vi "Actuators Jog Forward.vi"(0 "Notifier Name":string, 2 "Wait to Finish":bool, 5 "Channel":i32[](array[numeric]), 11 "Error In":errorcluster) -> (4 "Notifier Name Out":string, 15 "Error Out":errorcluster)   [LabVIEW 2020]
uses:
  Actuators Controls/Actuators Note Type.ctl
  Actuators Controls/Actuators Actions.ctl
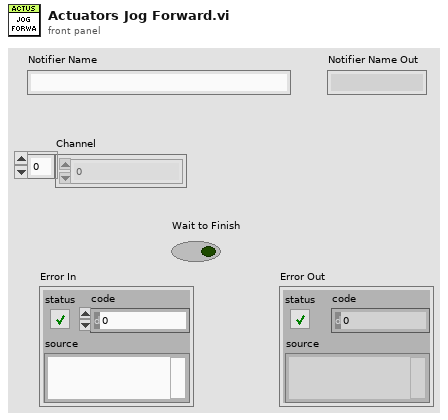
[diagram p1: front panel]
types:
  T1 = typedef "Actuators Note Type.ctl" = cluster{"Actions":T2, "Cmd Received ":bool, "Setpoint":dbl[], "Position":dbl[], "Channel":i32[], "Jog Step":dbl[], "Velocity":dbl[], "Acceleration":dbl[], "Status Bits":u32[], "Moving":bool[]}
  T2 = typedef "Actuators Actions.ctl" = enum16{"Nothing", "Get Position", "Get Acceleration", "Get Velocity", "Get Jog Step", "Set Acceleration", "Set Velocity", "Set Jog Step", "Move Absolute", "Move Relative", "Jog Forward", "Jog Reverse", "Halt", "Quit"}
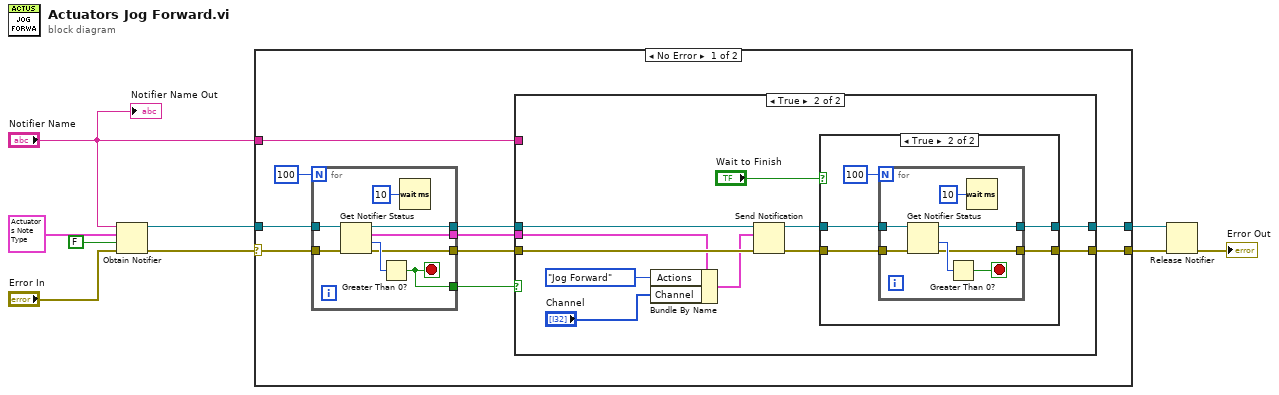
[diagram p0: block diagram]
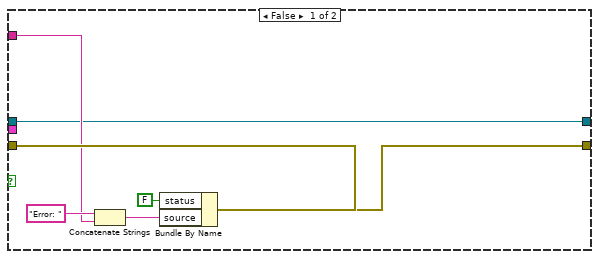
[diagram p2: hidden frame]
diagram:
  n1 = Obtain Notifier(name (unnamed)="Notifier Name", notification data type=T1 {"Actions"=enum."Nothing", "Cmd Received "=FALSE, "Setpoint"=[], "Position"=[], "Channel"=[], "Jog Step"=[], "Velocity"=[], "Acceleration"=[], "Status Bits"=[], "Moving"=[]} ("Actuators Note"), create if not found? (T)=FALSE, error in (no error)="Error In") -> (notifier out=w5:refnum<notifier>, error out=w8:errorcluster)  [unwired: 1 out]
  n2 = case shown="No Error" w8 {
    selector: w8 -> [w17 w60]
    tunnel: w5 -> [w18 w61]
    tunnel: "Notifier Name" -> [w12 _]
    tunnel: [w11 w61] -> w4
    tunnel: [w10 w60] -> w3
    frame No Error {
      n3 = for {
        N: 100 -> [_]
        tunnel: [w58] -> w14
        tunnel: w18 -> [w59]
        tunnel: [w57] -> w15
        tunnel: w17 -> [w54]
        tunnel: [w53] -> w16
        tunnel: [w52] -> w13
        stop <- w53 stop-if-true
        n4 = Get Notifier Status(notifier=w59, error in (no error)=w54) -> (notifier out=w57:refnum<notifier>, current notification=w58:T1, # waiting=w56:i32, error out=w52:errorcluster)  [unwired: 1 out]
        n5 = Greater Than 0?(x=w56) -> (x > 0?=w53:bool)
        n6 = Wait (ms)(milliseconds to wait=u32 10) -> ()  [unwired: 1 out]
      }
      n7 = case shown="True" w16 {
        tunnel: w15 -> [w21 w37]
        tunnel: w14 -> [_ w28]
        tunnel: w13 -> [w26 w36]
        tunnel: w12 -> [w22 _]
        tunnel: [w21 w32] -> w11
        tunnel: [w20 w33] -> w10
        frame False {
          n8 = Concatenate Strings("Error: " ("source"), w22) -> (w23:string)
          n9 = Bundle By Name(cluster=w26, "status"=FALSE, "source"=w23) -> (w20:errorcluster)
        }
        frame True {
          n10 = Bundle By Name(cluster=w28, "Actions"=Actuators_Actions."Jog Forward", "Channel"="Channel") -> (w29:T1)
          n11 = Send Notification(notification=w29, notifier=w37, error in (no error)=w36) -> (notifier out=w35:refnum<notifier>, error out=w34:errorcluster)
          n12 = case shown="True" "Wait to Finish" {
            tunnel: w35 -> [w39 w43]
            tunnel: w34 -> [w38 w42]
            tunnel: [w38 w41] -> w33
            tunnel: [w39 w40] -> w32
            frame False {
            }
            frame True {
              n13 = for {
                N: 100 -> [_]
                tunnel: w43 -> [w51]
                tunnel: [w50] -> w40
                tunnel: w42 -> [w47]
                tunnel: [w45] -> w41
                stop <- w46 stop-if-true
                n14 = Get Notifier Status(notifier=w51, error in (no error)=w47) -> (notifier out=w50:refnum<notifier>, # waiting=w49:i32, error out=w45:errorcluster)  [unwired: 2 out]
                n15 = Greater Than 0?(x=w49) -> (x > 0?=w46:bool)
                n16 = Wait (ms)(milliseconds to wait=u32 10) -> ()  [unwired: 1 out]
              }
            }
          }
        }
      }
    }
    frame Error {
    }
  }
  n17 = Release Notifier(notifier=w4, error in (no error)=w3) -> (error out=→"Error Out":errorcluster)  [unwired: 1 in, 2 out]
  "Notifier Name Out" <- "Notifier Name"
